vi "User Handling.vi"(6 "File In":string[](array[string]), 7 "Delete":bool, 8 "Add":bool, 9 "Name":string) -> (0 "File Out":string[](array[string]), 3 "Array":cluster{"String":string, "Numeric":dbl}[](array[cluster]))   [LabVIEW 2018]
panel:
  # "Outputs"
  # "Inputs"
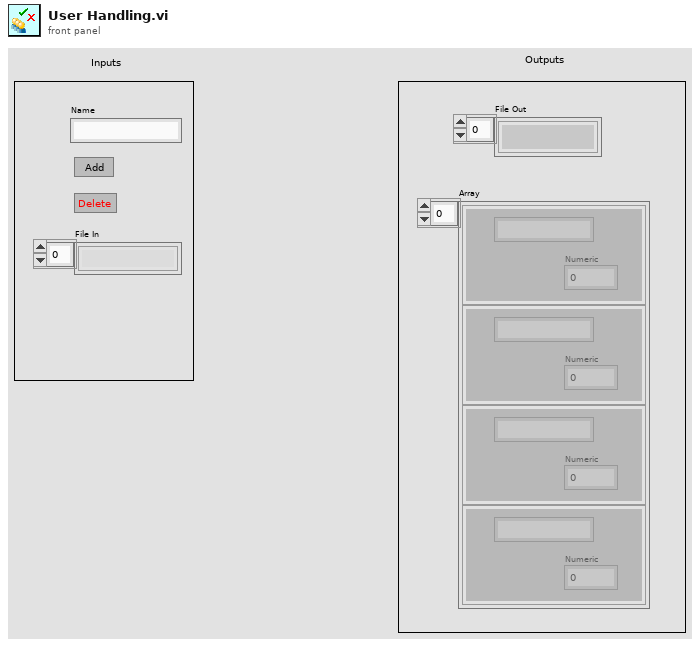
[diagram p1: front panel]
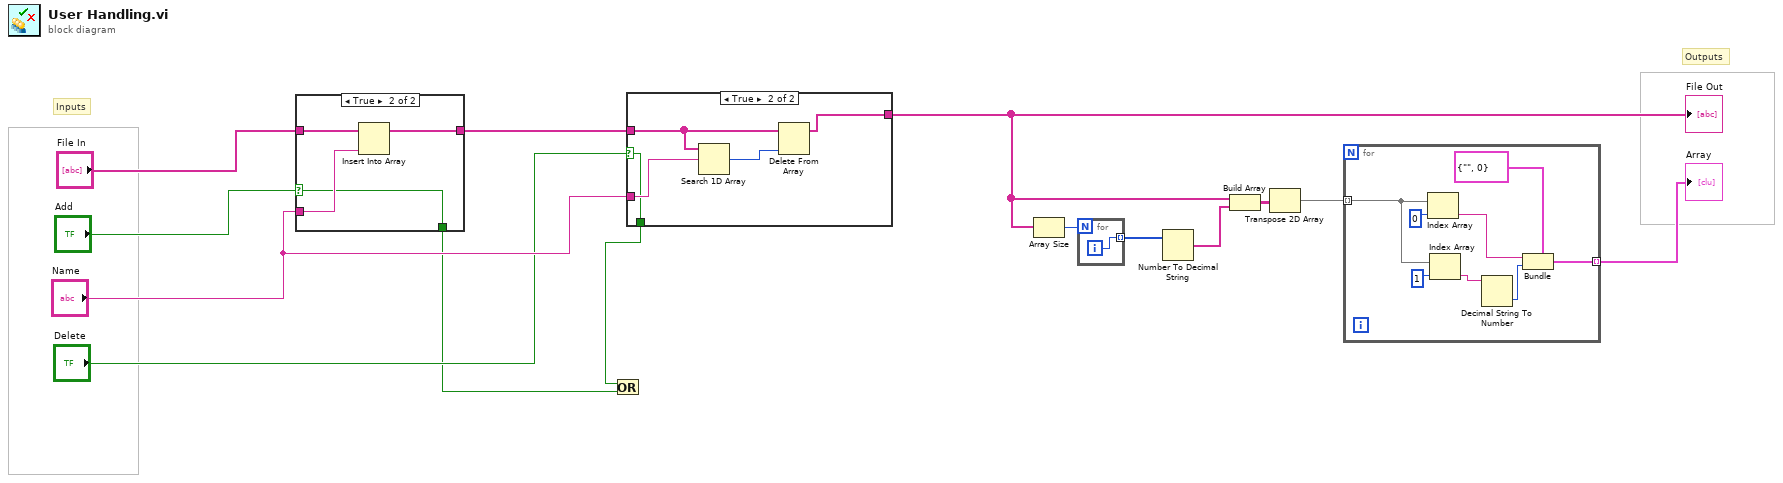
[diagram p0: block diagram]
diagram:
  # "Outputs"
  # "Inputs"
  n1 = case shown="True" "Add" {
    selector: "Add" -> [w15 w17]
    tunnel: "Name" -> [_ w20]
    tunnel: "File In" -> [w16 w19]
    tunnel: [w16 w18] -> w8
    tunnel: [w15 w17] -> w2
    frame False {
    }
    frame True {
      n2 = Insert Into Array(array=w19, new element=w20) -> (w18:string[])  [unwired: 1 in]
    }
  }
  n3 = case shown="True" "Delete" {
    selector: "Delete" -> [w21 w23]
    tunnel: w8 -> [w22 w27]
    tunnel: [w22 w26] -> w1
    tunnel: "Name" -> [_ w24]
    tunnel: [w21 w23] -> w3
    frame False {
    }
    frame True {
      n4 = Search 1D Array(1D array=w27, element=w24) -> (index of element=w25:i32)  [unwired: 1 in]
      n5 = Delete From Array(array=w27, index=w25) -> (array with subset deleted=w26:string[])  [unwired: 1 in, 1 out]
    }
  }
  "File Out" <- w1
  n6 = Or(x=w3, y=w2) -> ()  [unwired: 1 out]
  n7 = Array Size(array=w1) -> (size(s)=w14:i32)
  n8 = for {
    N: w14 -> [_]
    tunnel: [w28] -> w12 mode=indexing
    i -> [w28]
  }
  n9 = Number To Decimal String(number=w12) -> (decimal integer string=w13:string[])  [unwired: 1 in]
  n10 = Build Array(w1, w13) -> (w11:string[][])
  n11 = Transpose 2D Array(2D array=w11) -> (transposed array=w10:string[][])
  n12 = for {
    tunnel: w10 -> [w36] mode=indexing
    tunnel: [w29] -> w9 mode=indexing
    n13 = Index Array(array=w36, index=0) -> (element=w33:string)
    n14 = Index Array(array=w36, index=1) -> (element=w31:string)
    n15 = Decimal String To Number(string=w31) -> (number=w32:i32)  [unwired: 2 in, 1 out]
    n16 = Bundle(cluster=cluster{string, i32} {"", 0}, w33, w32) -> (w29:cluster{string, i32})
  }
  "Array" <- w9
